vi "Real Characteristic Polynomial.vi"(3 "Input Matrix":T1) -> (0 "error":i32, 1 "Characteristic Polynomial":dbl[](array[numeric]))   [LabVIEW 2020, in "NI_AALPro.lvlib"]
doc: "Computes the characteristic polynomial of <B>Input Matrix</B>. Wire data to the <B>Input Matrix</B> input to determine the polymorphic instance to use or manually select the instance."
uses:
  <vilib>/Analysis/NI_AALPro.lvlib
  <vilib>/Analysis/Matrix/Datatypes/RealMatrix.ctl
  <resource>/lvanlys.dll
  <vilib>/Analysis/Matrix/NI_Matrix.lvlib
panel:
  # "Real Matrix Characteristic Polynomial"
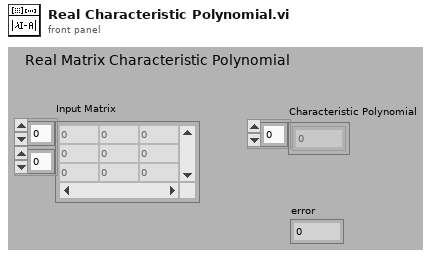
[diagram p1: front panel]
types:
  T1 = typedef "NI_Matrix.lvlib/RealMatrix.ctl" = dbl[][]
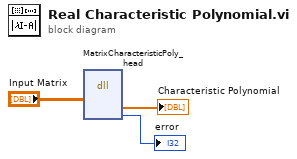
[diagram p0: block diagram]
diagram:
  n1 = dll-call lib="e:/builds/penguin/labview/branches/2020/dev/dist/resource/lvanlys.*" fn="MatrixCharacteristicPoly_head"("Input Matrix"="Input Matrix") -> ("Characteristic Polynomial"=→"Characteristic Polynomial":dbl[], "dsperr"=→"error":i32)  [unwired: 7 in, 2 out]
